vi "Serial Type to Data Bits.vi"(11 "serial type":T1) -> (3 "Data Bits":u32)   [LabVIEW 2015, in "Modbus Master System Explorer.lvlib"]
uses:
  Modbus Master System Explorer.lvlib
  Shared/Controls/Serial Type.ctl
  Shared/Modbus Master Shared.lvlib
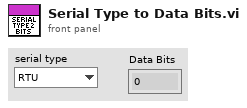
[diagram p1: front panel]
types:
  T1 = typedef "Modbus Master Shared.lvlib/Serial Type.ctl" = enum16{"RTU", "ASCII"}
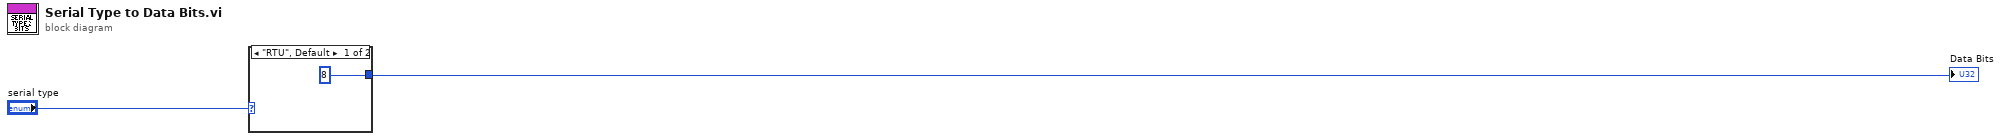
[diagram p0: block diagram]
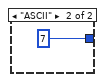
[diagram p2: hidden frame]
diagram:
  n1 = case shown="\"RTU\", Default" "serial type" {
    tunnel: [u32 8 ("Data Bits") u32 7 ("Data Bits")] -> w2
    frame "RTU", Default {
    }
    frame "ASCII" {
    }
  }
  "Data Bits" <- w2
